vi "DataEngine.vi"(8 "Op":T2(ring), 10 "Fips":i32[](array[numeric]), 11 "State":string) -> (0 "UpdateInfo":cluster{"time stamp":timestamp, i32}, 3 "Data":T1)   [LabVIEW 2017]
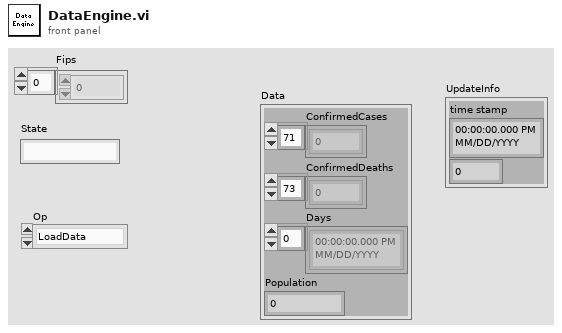
[diagram p1: front panel]
types:
  T1 = cluster{"ConfirmedCases":i32[], "ConfirmedDeaths":i32[], "Days":timestamp[], "Population":i32}
  T2 = enum16{"LoadData", "GetStateData", "GetCountyData", "GetCountyArray"}
  T3 = cluster{"Days":timestamp[], "CountyData":cluster{"CountyFips":i32, "StateFips/Pop":i32, "County":string, "State":string, "Cases":i32[]}[], "StateData":cluster{"CountyFips":i32, "StateFips":i32, "County":string, "State":string, "Cases":i32[]}[]}[]
  T4 = cluster{"Days":timestamp[], "CountyData":cluster{"CountyFips":i32, "StateFips/Pop":i32, "County":string, "State":string, "Cases":i32[]}[], "StateData":cluster{"CountyFips":i32, "StateFips":i32, "County":string, "State":string, "Cases":i32[]}[]}
  T5 = cluster{"CountyFips":i32, "StateFips":i32, "County":string, "State":string, "Cases":i32[]}[]
  T6 = cluster{"CountyFips":i32, "StateFips/Pop":i32, "County":string, "State":string, "Cases":i32[]}[]
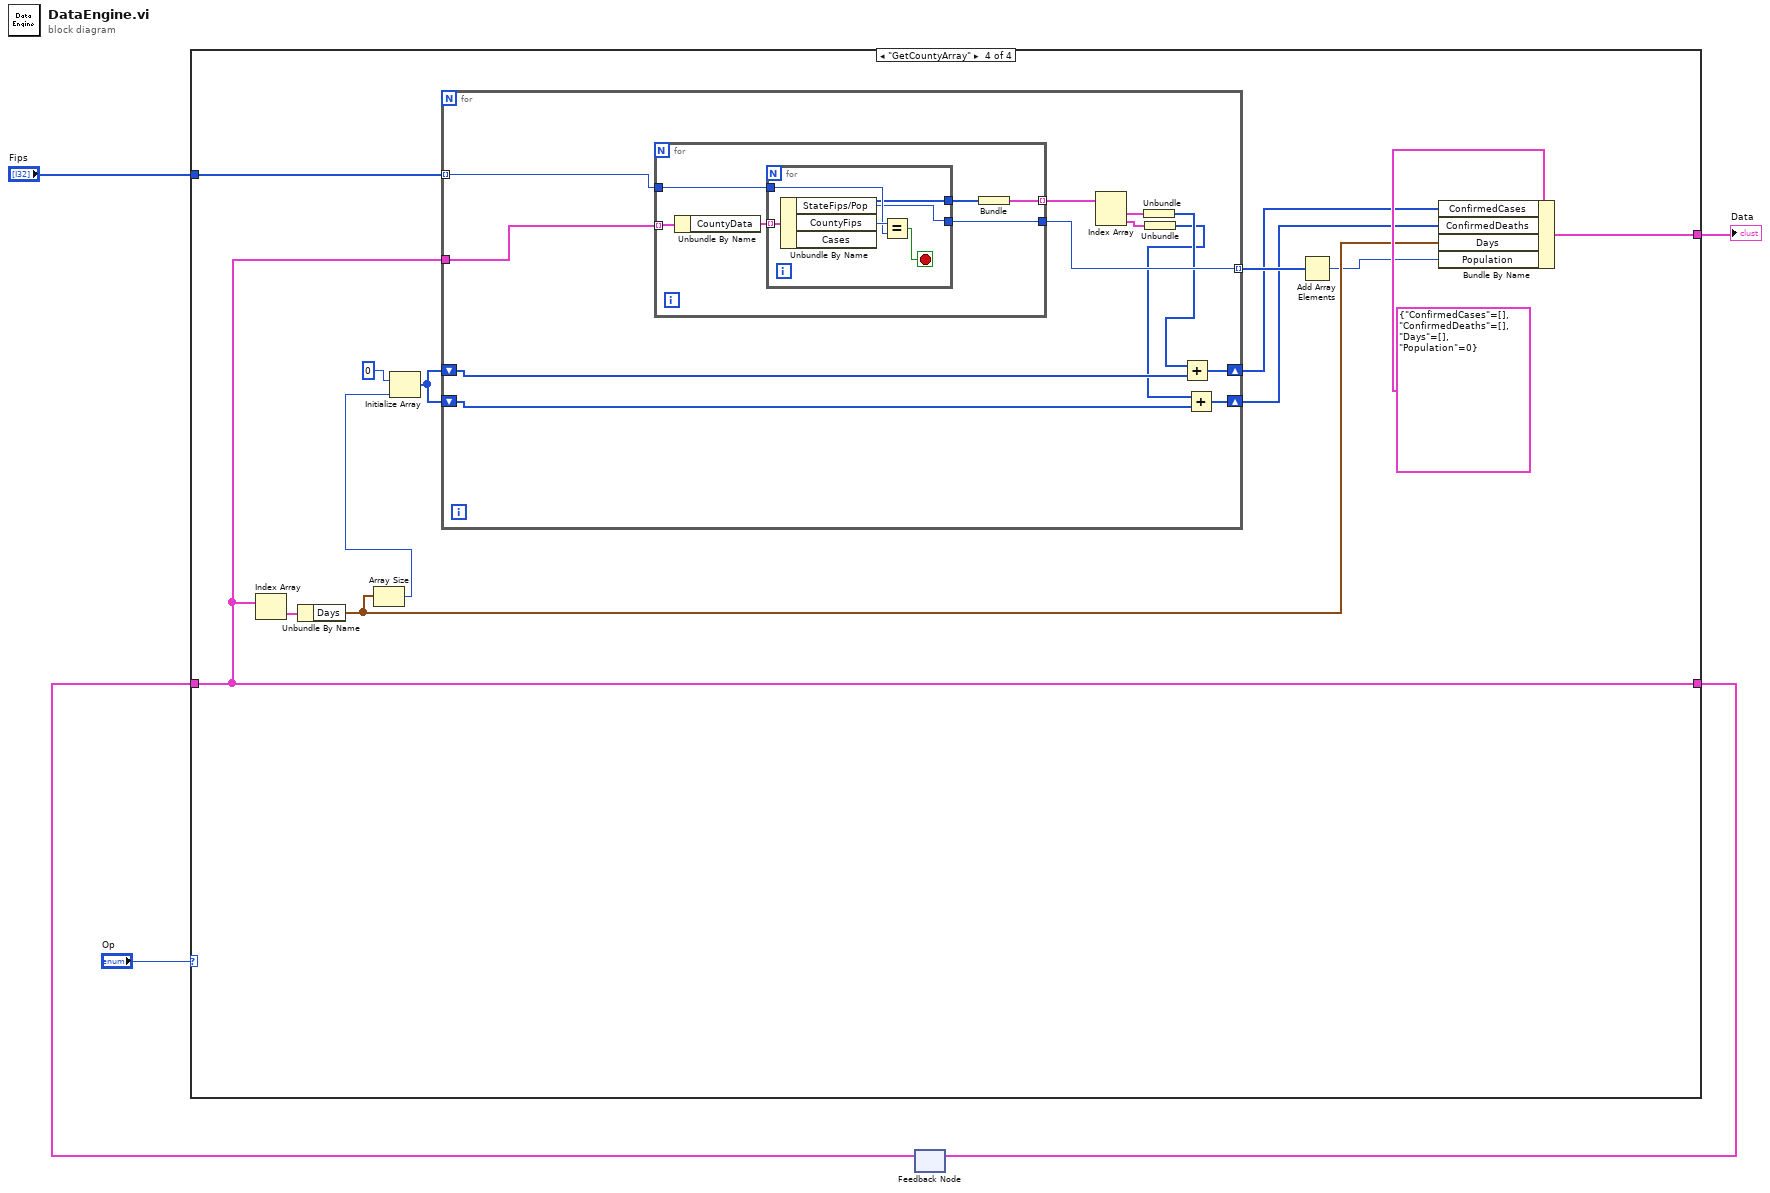
[diagram p0: block diagram]
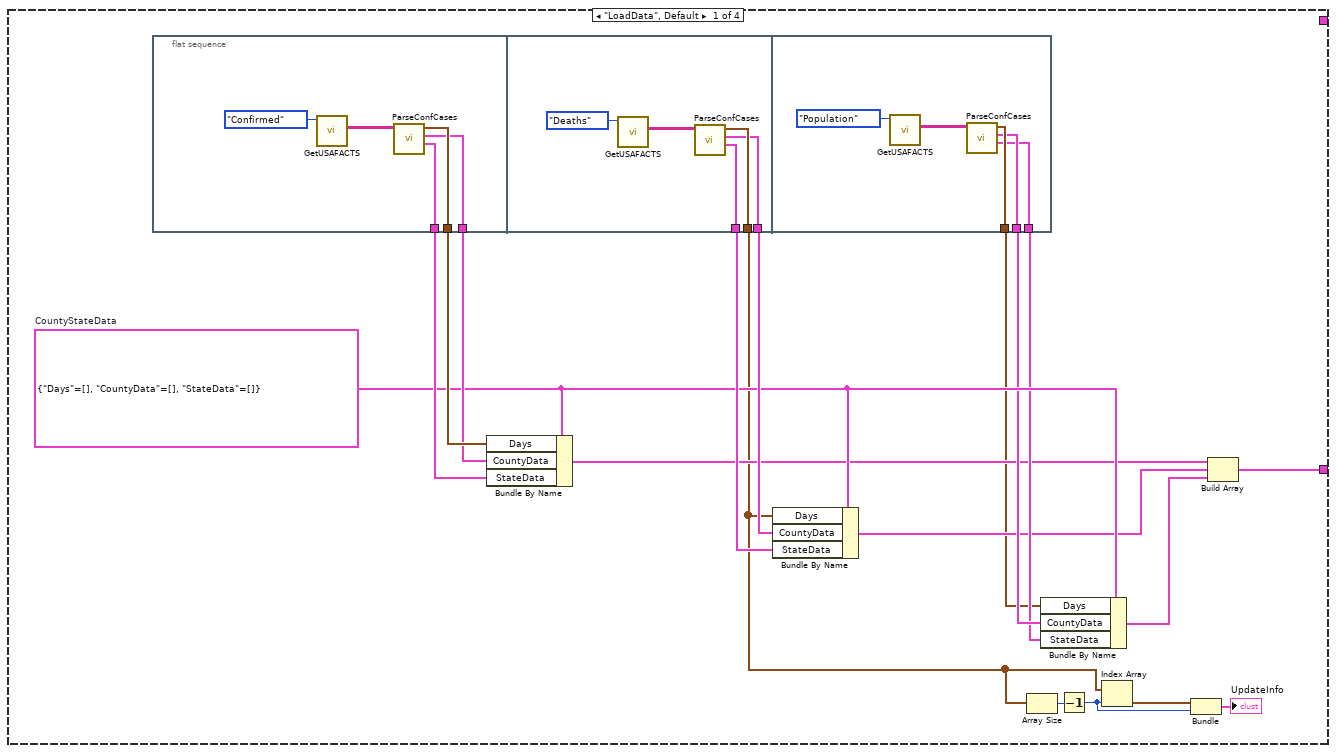
[diagram p2: hidden frame]
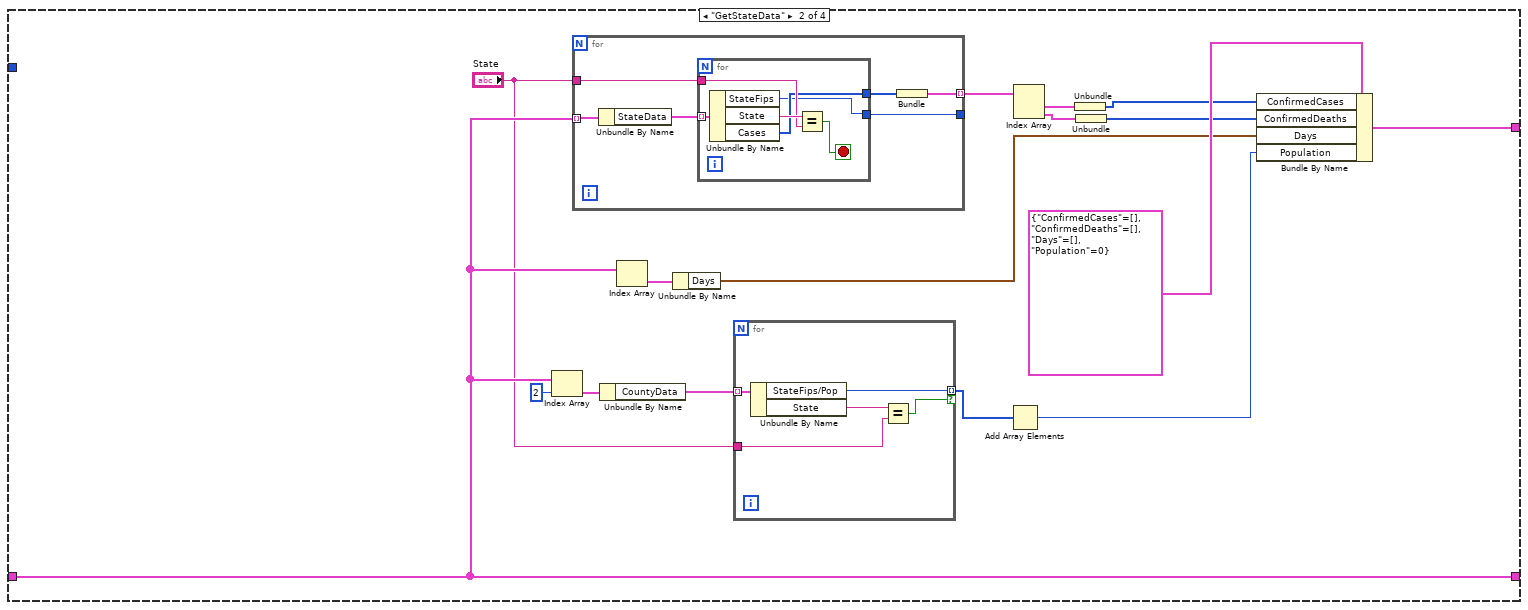
[diagram p3: hidden frame]
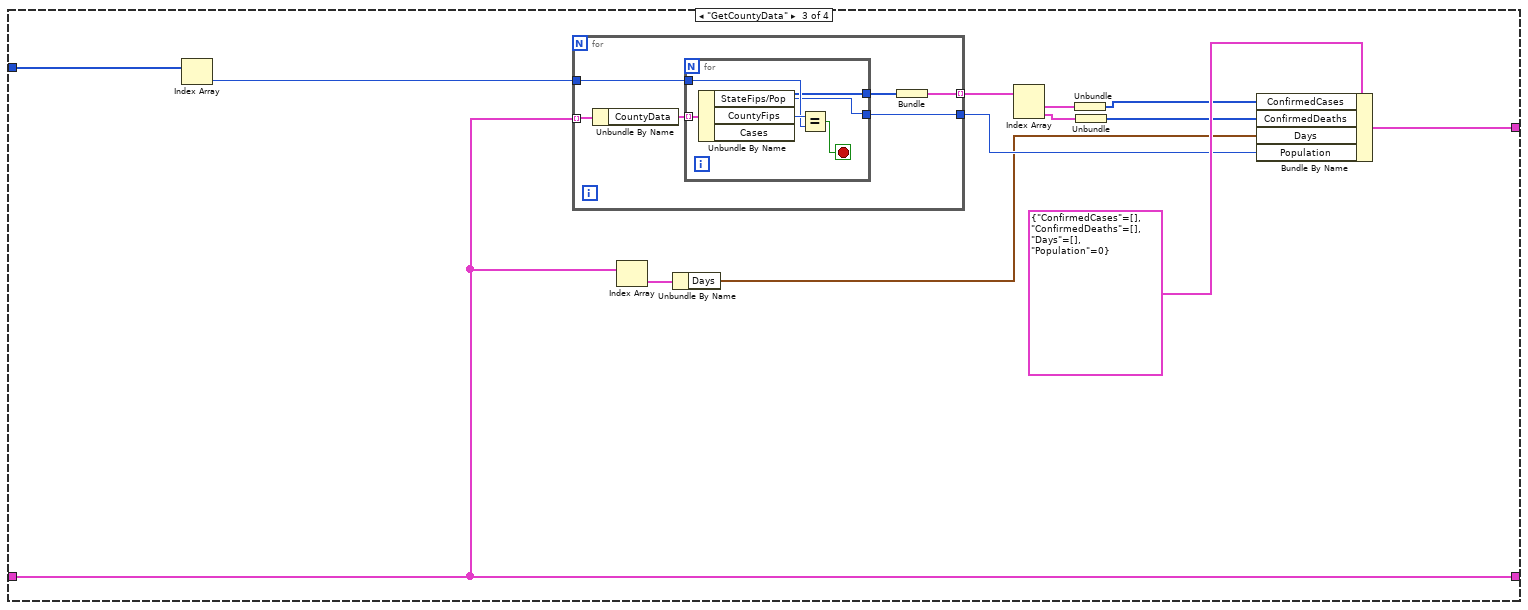
[diagram p4: hidden frame]
diagram:
  n1 = feedback #1() -> (w3:T3)  [unwired: 1 in]
  n2 = case shown="\"GetCountyArray\"" "Op" {
    tunnel: [w12 w45 w77 w106] -> w4
    tunnel: w3 -> [_ w45 w77 w106]
    tunnel: [_ w46 w74 w108] -> w2
    tunnel: "Fips" -> [_ _ w73 w107]
    frame "LoadData", Default {
      w18 = T4 {"Days"=[], "CountyData"=[], "StateData"=[]}  # CountyStateData
      n3 = flat-sequence {
        tunnel: [w26] -> w23
        tunnel: [w25] -> w22
        tunnel: [w24] -> w21
        tunnel: [w31] -> w6
        tunnel: [w30] -> w20
        tunnel: [w29] -> w19
        tunnel: [w36] -> w11
        tunnel: [w35] -> w17
        tunnel: [w34] -> w16
        frame #0 {
          n4 = call "GetUSAFACTS.vi"("index"=enum16{"Confirmed", "Deaths", "Population"}."Confirmed") -> ("Data"=w27:string[][])  [unwired: 9 in, 1 out]
          n5 = call "ParseConfCases.vi"("DataIn"=w27) -> ("StateData"=w24:T5, "CountyData"=w25:T6, "Days"=w26:timestamp[])  [unwired: 8 in]
        }
        frame #1 {
          n6 = call "GetUSAFACTS.vi"("index"=enum16{"Confirmed", "Deaths", "Population"}."Deaths") -> ("Data"=w33:string[][])  [unwired: 9 in, 1 out]
          n7 = call "ParseConfCases.vi"("DataIn"=w33) -> ("StateData"=w29:T5, "CountyData"=w30:T6, "Days"=w31:timestamp[])  [unwired: 8 in]
        }
        frame #2 {
          n8 = call "GetUSAFACTS.vi"("index"=enum16{"Confirmed", "Deaths", "Population"}."Population") -> ("Data"=w37:string[][])  [unwired: 9 in, 1 out]
          n9 = call "ParseConfCases.vi"("DataIn"=w37) -> ("StateData"=w34:T5, "CountyData"=w35:T6, "Days"=w36:timestamp[])  [unwired: 8 in]
        }
      }
      n10 = Bundle By Name(cluster=w18, "Days"=w23, "CountyData"=w22, "StateData"=w21) -> (w15:T4)
      n11 = Bundle By Name(cluster=w18, "Days"=w6, "CountyData"=w20, "StateData"=w19) -> (w14:T4)
      n12 = Array Size(array=w6) -> (size(s)=w10:i32)
      n13 = Bundle By Name(cluster=w18, "Days"=w11, "CountyData"=w17, "StateData"=w16) -> (w13:T4)
      n14 = Decrement(x=w10) -> (x-1=w8:i32)
      n15 = Index Array(array=w6, index=w8) -> (element=w9:timestamp)
      n16 = Bundle("time stamp"=w9, w8) -> (→"UpdateInfo":cluster{"time stamp":timestamp, i32})  [unwired: 1 in]
      n17 = Build Array(w15, w14, w13) -> (w12:T3)
    }
    frame "GetStateData" {
      n18 = Index Array(array=w45, index=2) -> (element=w43:T4)
      n19 = for {
        tunnel: w45 -> [w65] mode=indexing
        tunnel: "State" -> [w63]
        tunnel: [w61] -> w54 mode=indexing
        tunnel: [w60] -> _
        n20 = Unbundle By Name(w65) -> ("StateData"=w64:T5)
        n21 = for {
          tunnel: w64 -> [w68] mode=indexing
          tunnel: w63 -> [w70]
          tunnel: [w67] -> w62
          tunnel: [w66] -> w60
          stop <- w69 stop-if-true
          n22 = Unbundle By Name(w68) -> ("StateFips"=w66:i32, "State"=w71:string, "Cases"=w67:i32[])
          n23 = Equal?(x=w71, y=w70) -> (x = y?=w69:bool)
        }
        n24 = Bundle("Cases"=w62) -> (w61:cluster{"Cases":i32[]})  [unwired: 1 in]
      }
      n25 = Unbundle By Name(w43) -> ("CountyData"=w42:T6)
      n26 = Index Array(array=w45) -> (element=w48:T4)  [unwired: 1 in]
      n27 = Unbundle By Name(w48) -> ("Days"=w47:timestamp[])
      n28 = for {
        tunnel: w42 -> [w59] mode=indexing
        tunnel: "State" -> [w57]
        tunnel: [w56] -> w40 mode=indexing if=w55
        n29 = Unbundle By Name(w59) -> ("StateFips/Pop"=w56:i32, "State"=w58:string)
        n30 = Equal?(x=w58, y=w57) -> (x = y?=w55:bool)
      }
      n31 = Add Array Elements(numeric array=w40) -> (sum=w39:i32)
      n32 = Index Array(array=w54) -> (element #1=w53:cluster{"Cases":i32[]}, element #2=w52:cluster{"Cases":i32[]})  [unwired: 2 in]
      n33 = Unbundle(w53) -> ("Cases"=w50:i32[])
      n34 = Unbundle(w52) -> ("Cases"=w49:i32[])
      n35 = Bundle By Name(cluster=T1 {"ConfirmedCases"=[], "ConfirmedDeaths"=[], "Days"=[], "Population"=0}, "ConfirmedCases"=w50, "ConfirmedDeaths"=w49, "Days"=w47, "Population"=w39) -> (w46:T1)
    }
    frame "GetCountyData" {
      n36 = Index Array(array=w73) -> (element=w72:i32)  [unwired: 1 in]
      n37 = for {
        tunnel: w77 -> [w90] mode=indexing
        tunnel: w72 -> [w88]
        tunnel: [w86] -> w84 mode=indexing
        tunnel: [w85] -> w78
        n38 = Unbundle By Name(w90) -> ("CountyData"=w89:T6)
        n39 = for {
          tunnel: w89 -> [w93] mode=indexing
          tunnel: w88 -> [w95]
          tunnel: [w92] -> w87
          tunnel: [w91] -> w85
          stop <- w94 stop-if-true
          n40 = Unbundle By Name(w93) -> ("StateFips/Pop"=w91:i32, "CountyFips"=w96:i32, "Cases"=w92:i32[])
          n41 = Equal?(x=w96, y=w95) -> (x = y?=w94:bool)
        }
        n42 = Bundle("Cases"=w87) -> (w86:cluster{"Cases":i32[]})  [unwired: 1 in]
      }
      n43 = Index Array(array=w77) -> (element=w76:T4)  [unwired: 1 in]
      n44 = Unbundle By Name(w76) -> ("Days"=w75:timestamp[])
      n45 = Index Array(array=w84) -> (element #1=w83:cluster{"Cases":i32[]}, element #2=w82:cluster{"Cases":i32[]})  [unwired: 2 in]
      n46 = Unbundle(w83) -> ("Cases"=w80:i32[])
      n47 = Unbundle(w82) -> ("Cases"=w79:i32[])
      n48 = Bundle By Name(cluster=T1 {"ConfirmedCases"=[], "ConfirmedDeaths"=[], "Days"=[], "Population"=0}, "ConfirmedCases"=w80, "ConfirmedDeaths"=w79, "Days"=w75, "Population"=w78) -> (w74:T1)
    }
    frame "GetCountyArray" {
      n49 = Index Array(array=w106) -> (element=w104:T4)  [unwired: 1 in]
      n50 = Unbundle By Name(w104) -> ("Days"=w103:timestamp[])
      n51 = Array Size(array=w103) -> (size(s)=w97:i32)
      n52 = Initialize Array(0, w97) -> (w102:i32[])
      n53 = for {
        tunnel: w107 -> [w118] mode=indexing
        tunnel: w106 -> [w117]
        tunnel: [w116] -> w105 mode=indexing
        shift-right: [w113] -> w101
        shift-left: w102 -> [w115]
        shift-right: [w110] -> w99
        shift-left: w102 -> [w112]
        n54 = for {
          tunnel: w117 -> [w127] mode=indexing
          tunnel: w118 -> [w125]
          tunnel: [w123] -> w121 mode=indexing
          tunnel: [w122] -> w116
          n55 = Unbundle By Name(w127) -> ("CountyData"=w126:T6)
          n56 = for {
            tunnel: w126 -> [w130] mode=indexing
            tunnel: w125 -> [w132]
            tunnel: [w129] -> w124
            tunnel: [w128] -> w122
            stop <- w131 stop-if-true
            n57 = Unbundle By Name(w130) -> ("StateFips/Pop"=w128:i32, "CountyFips"=w133:i32, "Cases"=w129:i32[])
            n58 = Equal?(x=w133, y=w132) -> (x = y?=w131:bool)
          }
          n59 = Bundle("Cases"=w124) -> (w123:cluster{"Cases":i32[]})  [unwired: 1 in]
        }
        n60 = Index Array(array=w121) -> (element #1=w120:cluster{"Cases":i32[]}, element #2=w119:cluster{"Cases":i32[]})  [unwired: 2 in]
        n61 = Unbundle(w120) -> ("Cases"=w114:i32[])
        n62 = Unbundle(w119) -> ("Cases"=w111:i32[])
        n63 = Add(x=w114, y=w115) -> (x+y=w113:i32[])
        n64 = Add(x=w111, y=w112) -> (x+y=w110:i32[])
      }
      n65 = Add Array Elements(numeric array=w105) -> (sum=w100:i32)
      n66 = Bundle By Name(cluster=T1 {"ConfirmedCases"=[], "ConfirmedDeaths"=[], "Days"=[], "Population"=0}, "ConfirmedCases"=w101, "ConfirmedDeaths"=w99, "Days"=w103, "Population"=w100) -> (w108:T1)
    }
  }
  "Data" <- w2
  n67 = feedback-in #1(w4) -> ()
